vi "Rinocloud_real-time_monitoring2.vi"() -> ()   [LabVIEW 2013]
uses:
  Rinocloud_global_variable.vi
  Rinocloud API endpoint VIs/API_endpoint_subVIs/Rinocloud_get_metadata_field_value_subVIs/get_string_value.vi
panel:
  out "System Waveform Graph":dbl[](graph)
  out "Data chunk":string
  in  "Start append":bool
  in  "Record name":string
  in  "create empty":bool
  in  "Request period (s)":dbl
  out "Status:":string="OFF"
  in  "stop":bool
  out "Parent folder:":string
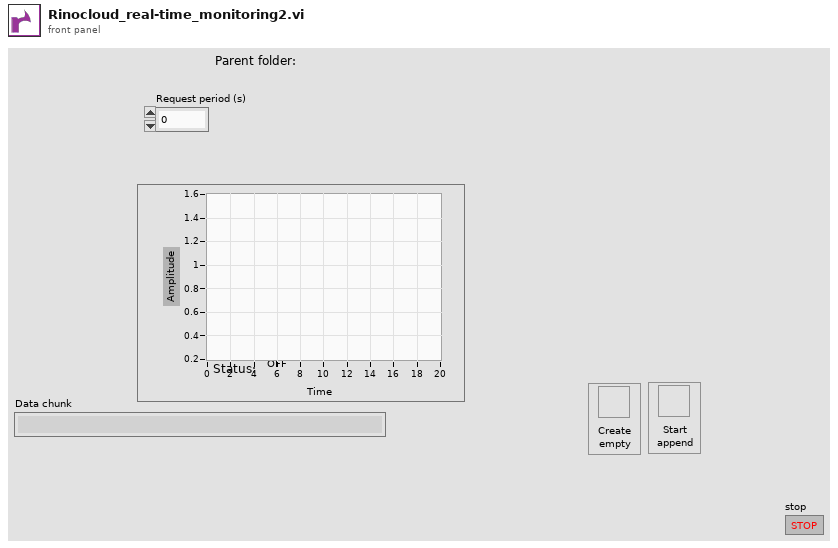
[diagram p1: front panel]
types:
  T1 = cluster{"Record ID":string, "Status":string, "Record name":string, "Parent ID":string, "Request period (s)":dbl, "Sending...":bool, "Parent folder":string, "HTTP resp body":string, "Data chunk":string, "error out":errorcluster, "error in (no error)":errorcluster, "x array":dbl, "y array":dbl[]}
  T2 = enum16{"initialize", "create empty", "append", "wait for event", "start append"}
  T3 = enum8{"Enabled", "Disabled", "Disabled and Grayed Out"}
  T4 = enum16{"initialize", "create empty", "append", "wait for event"}
  T5 = enum16{"Numeric", "String", "1D array of strings", "1D array of doubles", "Data JSON string", "<null>"}
  T6 = cluster{"Attribute":string, "Value":string, "Data type":enum16{"Numeric", "String", "1D array of strings", "1D array of doubles", "Data JSON string", "<null>"}}
  T7 = cluster{"Attribute":string, "Value":string, "Data type":enum16{"Numeric", "String", "1D array of strings", "1D array of doubles", "Data JSON string", "<null>"}}[]
  T8 = cluster{"headers":string, "body":string, "ID":string, "Saved":bool}
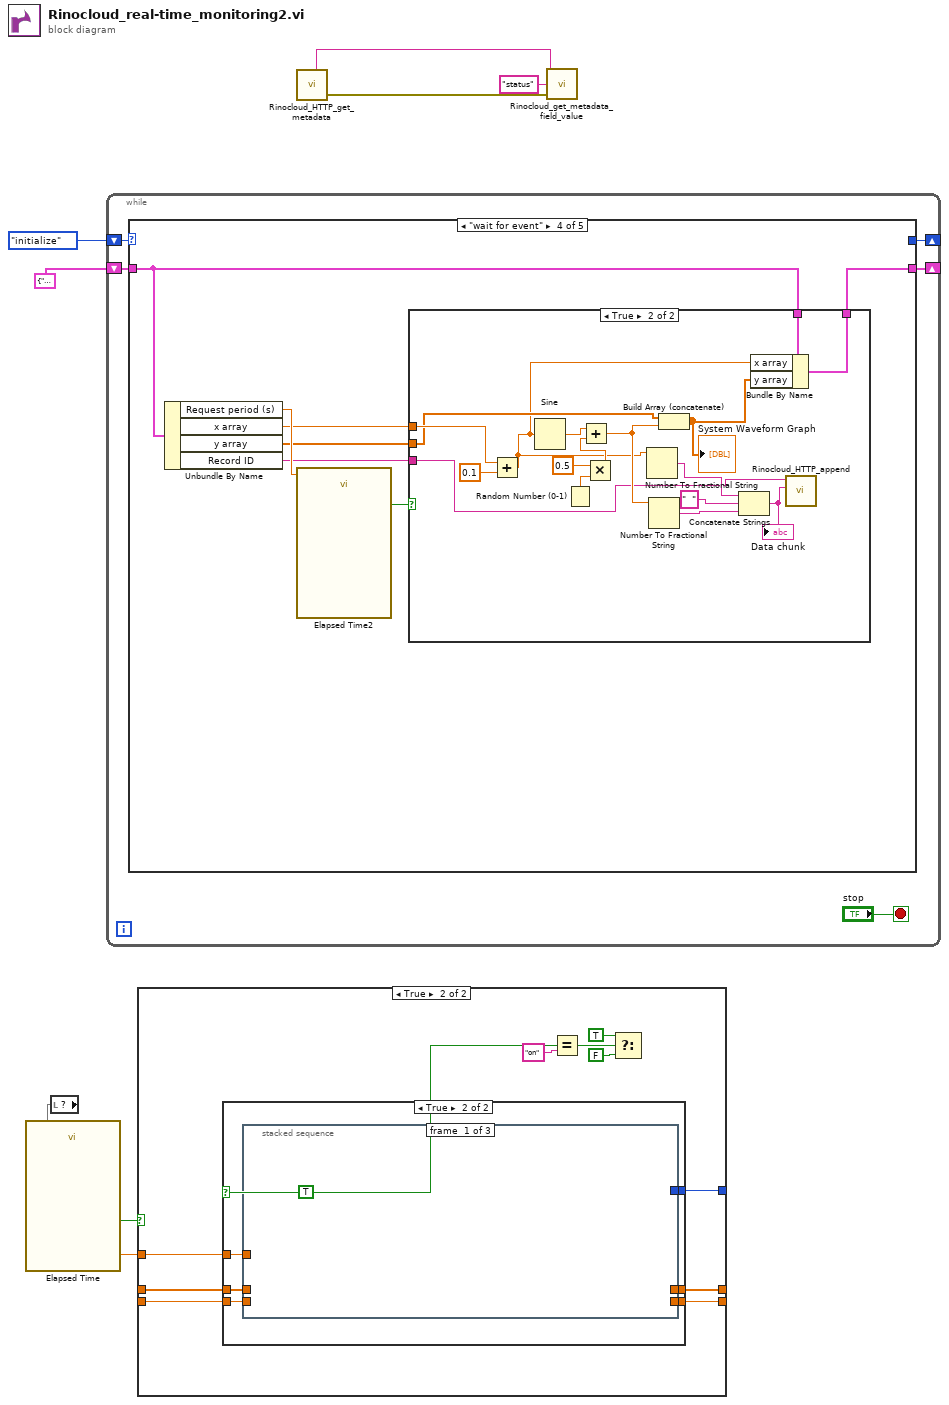
[diagram p0: block diagram]
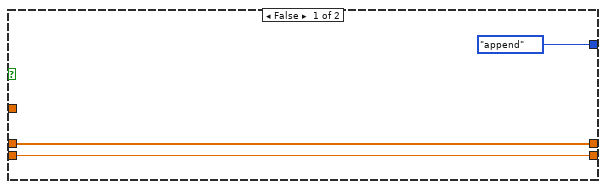
[diagram p2: hidden frame]
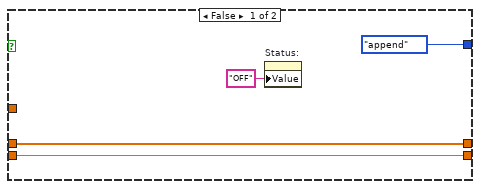
[diagram p3: hidden frame]
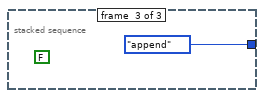
[diagram p5: hidden frame]
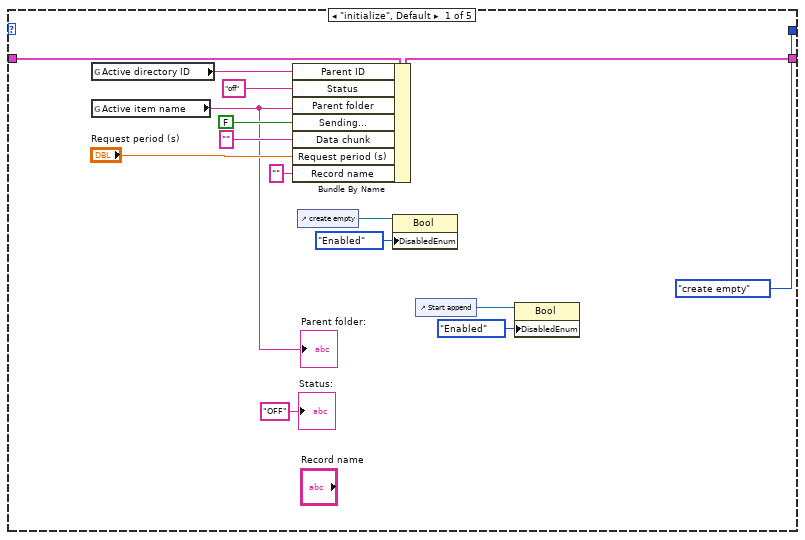
[diagram p6: hidden frame]
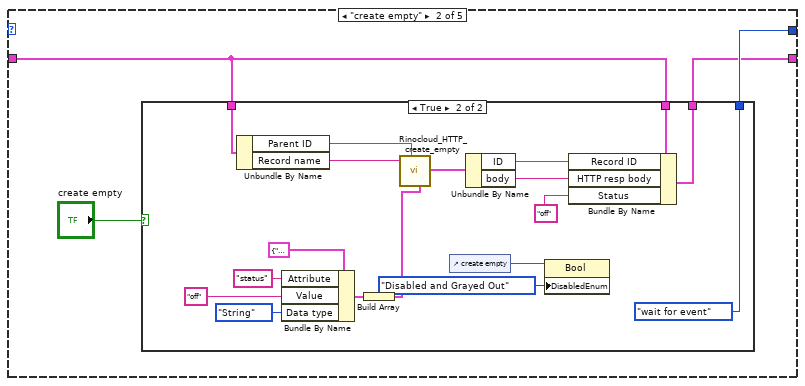
[diagram p7: hidden frame]
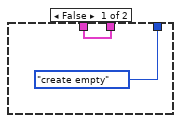
[diagram p8: hidden frame]
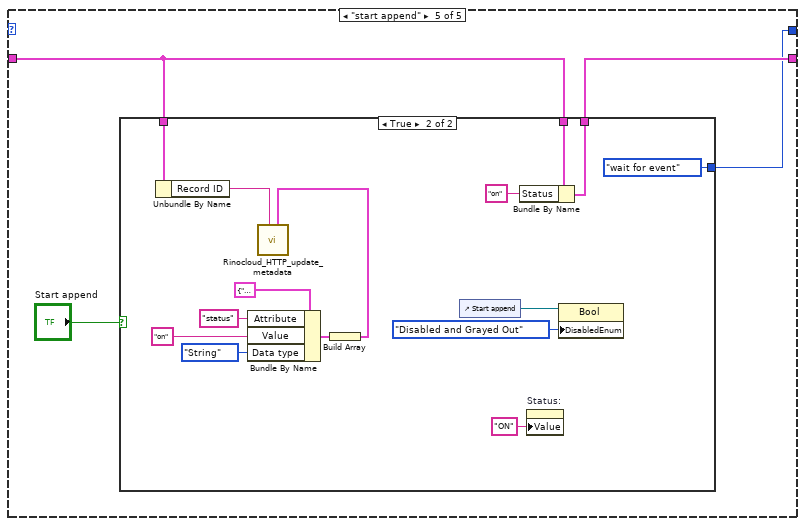
[diagram p11: hidden frame]
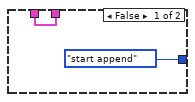
[diagram p12: hidden frame]
diagram:
  n1 = local read item#-1() -> (w7)
  n2 = call "Elapsed Time"("Time Target (s)"=w7) -> ("Present (s)"=w9:dbl, "Time has Elapsed"=w6:bool)  [unwired: 11 in, 6 out]
  n3 = while {
    shift-right: [w14] -> _
    shift-left: T2."initialize" -> [w15]
    shift-right: [w16] -> _
    shift-left: T1 {"Record ID"="", "Status"="", "Record name"="", "Parent ID"="", "Request period (s)"=1.0, "Sending..."=FALSE, "Parent folder"="", "HTTP resp body"="", "Data chunk"="", "error out"={"status"=FALSE, "code"=0, "source"=""}, "error in (no error)"={"status"=FALSE, "code"=0, "source"=""}, "x array"=0.0, "y array"=[]} ("Cluster") -> [w17]
    stop <- "stop" stop-if-true
    n4 = case shown="\"wait for event\"" w15 {
      tunnel: [w32 w34 _ w59 w83] -> w16
      tunnel: w17 -> [w33 w35 _ w60 w84]
      tunnel: [T4."create empty" w37 _ _ w82] -> w14
      frame "initialize", Default {
        n5 = global read "Rinocloud_global_variable.vi" "Active directory ID"() -> (w30:string)
        n6 = global read "Rinocloud_global_variable.vi" "Active item name"() -> (w26:string)
        "Parent folder:" <- w26
        n7 = Bundle By Name(cluster=w33, "Parent ID"=w30, "Status"="off", "Parent folder"=w26, "Sending..."=FALSE, "Data chunk"="", "Request period (s)"="Request period (s)", "Record name"="") -> (w32:T1)
        n8 = control-ref of="create empty"() -> (w23:refnum<vi>)
        n9 = property class="Bool"(reference=w23, "DisabledEnum"=T3."Enabled" ("Disabled")) -> ()  [unwired: 1 in, 2 out]
        n10 = control-ref of="Start append"() -> (w19:refnum<vi>)
        n11 = property class="Bool"(reference=w19, "DisabledEnum"=T3."Enabled" ("Disabled")) -> ()  [unwired: 1 in, 2 out]
        "Status:" <- "OFF" ("Status:")
      }
      frame "create empty" {
        n12 = case shown="True" "create empty" {
          tunnel: [T4."create empty" T4."wait for event"] -> w37
          tunnel: w35 -> [_ w49]
          tunnel: w35 -> [w38 w46]
          tunnel: [w38 w45] -> w34
          frame False {
          }
          frame True {
            n13 = Unbundle By Name(w49) -> ("Parent ID"=w48:string, "Record name"=w47:string)
            n14 = Bundle By Name(cluster=T6 {"Attribute"="", "Value"="", "Data type"=enum."<null>"} ("extra information field 4"), "Attribute"="status", "Value"="off", "Data type"=T5."String") -> (w53:T6)
            n15 = Build Array(w53) -> (w52:T7)
            n16 = call "Rinocloud_HTTP_create_empty.vi"("Extra metadata array"=w52, "Parent ID"=w48, "Name"=w47) -> ("Status"=w51:T8)  [unwired: 5 in, 1 out]
            n17 = control-ref of="create empty"() -> (w41:refnum<vi>)
            n18 = Unbundle By Name(w51) -> ("ID"=w44:string, "body"=w43:string)
            n19 = property class="Bool"(reference=w41, "DisabledEnum"=T3."Disabled and Grayed Out" ("Disabled")) -> ()  [unwired: 1 in, 2 out]
            n20 = Bundle By Name(cluster=w46, "Record ID"=w44, "HTTP resp body"=w43, "Status"="off" ("Status:")) -> (w45:T1)
          }
        }
      }
      frame "append" {
      }
      frame "wait for event" {
        n21 = Unbundle By Name(w60) -> ("Request period (s)"=w64:dbl, "x array"=w61:dbl, "y array"=w62:dbl[], "Record ID"=w58:string)
        n22 = call "Elapsed Time2"("Time Target (s)"=w64) -> ("Time has Elapsed"=w63:bool)  [unwired: 11 in, 7 out]
        n23 = case shown="True" w63 {
          tunnel: w62 -> [_ w70]
          tunnel: w61 -> [_ w71]
          tunnel: w60 -> [_ w69]
          tunnel: [_ w66] -> w59
          tunnel: w58 -> [_ w65]
          frame False {
          }
          frame True {
            n24 = Add(x=w71, y=0.1) -> (x+y=w68:dbl)
            n25 = Sine(x=w68) -> (sin(x)=w75:dbl)
            n26 = Random Number (0-1)() -> (number: 0 to 1=w77:dbl)
            n27 = Multiply(x=0.5, y=w77) -> (x*y=w74:dbl)
            n28 = Add(x=w75, y=w74) -> (x+y=w73:dbl)
            n29 = Number To Fractional String(number=w68) -> (F-format string=w78:string)  [unwired: 3 in]
            n30 = Number To Fractional String(number=w73) -> (F-format string=w81:string)  [unwired: 3 in]
            n31 = Build Array (concatenate)(w70, w73) -> (w67:dbl[])
            "System Waveform Graph" <- w67
            n32 = Concatenate Strings(w78, "  " ("string"), w81) -> (w72:string)
            "Data chunk" <- w72
            n33 = Bundle By Name(cluster=w69, "x array"=w68, "y array"=w67) -> (w66:T1)
            n34 = call "Rinocloud_HTTP_append.vi"("chunk"=w72, "ID"=w65) -> ()  [unwired: 4 in, 3 out]
          }
        }
      }
      frame "start append" {
        n35 = case shown="True" "Start append" {
          tunnel: w84 -> [_ w102]
          tunnel: w84 -> [w87 w92]
          tunnel: [w87 w89] -> w83
          tunnel: [T2."start append" T2."wait for event"] -> w82
          frame False {
          }
          frame True {
            n36 = Unbundle By Name(w102) -> ("Record ID"=w101:string)
            n37 = Bundle By Name(cluster=T6 {"Attribute"="", "Value"="", "Data type"=enum."<null>"} ("extra information field 4"), "Attribute"="status", "Value"="on", "Data type"=T5."String") -> (w96:T6)
            n38 = Build Array(w96) -> (w95:T7)
            n39 = call "Rinocloud_HTTP_update_metadata.vi"("Extra metadata array"=w95, "self ID"=w101) -> ()  [unwired: 8 in, 2 out]
            n40 = control-ref of="Start append"() -> (w93:refnum<vi>)
            n41 = Bundle By Name(cluster=w92, "Status"="on") -> (w89:T1)
            n42 = property on="Status:" class="Str"("Value"="ON" ("Status:")) -> ()  [unwired: 2 in, 2 out]
            n43 = property class="Bool"(reference=w93, "DisabledEnum"=T3."Disabled and Grayed Out" ("Disabled")) -> ()  [unwired: 1 in, 2 out]
          }
        }
      }
    }
  }
  n44 = case shown="True" w6 {
    tunnel: [enum16{"initialize", "append", "pause"}."append" w117] -> w8
    tunnel: w9 -> [_ w116]
    tunnel: [w104 w110] -> w10
    tunnel: [w104 w109] -> w11
    tunnel: [w103 w108] -> w12
    tunnel: [w103 w107] -> w13
    frame False {
    }
    frame True {
      n45 = Equal?(y="on") -> (x=w106:string, x = y?=w114:bool)
      n46 = Select(t=TRUE, s=w114, f=FALSE) -> (s? t:f=w111:bool)
      n47 = case shown="True" w111 {
        tunnel: [enum16{"initialize", "append", "pause"}."append" w127] -> w117
        tunnel: w116 -> [_ w126]
        tunnel: w110 -> [w119 w125]
        tunnel: [w119 w124] -> w109
        tunnel: w108 -> [w118 w123]
        tunnel: [w118 w122] -> w107
        frame False {
          n48 = property on="Status:" class="Str"("Value"="OFF" ("Status:")) -> ()  [unwired: 2 in, 2 out]
        }
        frame True {
          n49 = stacked-sequence {
            tunnel: [_ _ enum16{"initialize", "append", "pause"}."append"] -> w127
            tunnel: w126 -> [_ _ _]
            tunnel: w125 -> [_ _ _]
            tunnel: [_ w129 _] -> w124
            tunnel: w123 -> [_ _ _]
            tunnel: [_ _ _] -> w122
            frame #0 {
              w128 = TRUE ("Sending...")
            }
            frame #1 {
            }
            frame #2 {
              w131 = FALSE ("Sending...")
            }
          }
        }
      }
    }
  }
  n50 = call "Rinocloud_HTTP_get_metadata.vi"() -> ("error out"=w2:errorcluster, "metadata (JSON)"=w4:string)  [unwired: 5 in, 5 out]
  n51 = call-poly "Rinocloud_get_metadata_field_value.vi"("error in (no error)"=w2, "field name"="status" ("Parameter Name"), "metadata JSON string"=w4) -> ()  [unwired: 1 in, 2 out]
